vi "stage-controller.vi"() -> ()   [LabVIEW 2014]
uses:
  Stage SubVis/Move stage command - Global - SubVI.ctl
  Stage SubVis/user event out globals - SubVI.vi
  lib/Madlib/Madlib.lvlib
panel:
  out "Current Z (um)":ext
  out "Current Y (um)":ext
  out "Current X (um)":ext
  in  "Curr. Z":dbl(slide) scale=0.0..1.0
  out "Current (X,Y)":cluster{ext[], ext[]}(graph)
  out "At limit 3":bool
  out "At limit 2":bool
  out "At limit":bool
  in  "x,y step (um)":ext=10.0 format="%_5g"
  in  "z step (um)":ext=0.1 format="%_5g"
  in  "y-":bool
  in  "x-":bool
  in  "x+":bool
  in  "z-":bool
  in  "z+":bool
  in  "y+":bool
  in  "Reset stage to center\n         (x, y, and z)":bool
  in  "Stop":bool
  out "Z Range (um)":dbl format="%#_13g"
  out "Y Range (um)":dbl format="%#_13g"
  out "X Range (um)":dbl format="%#_13g"
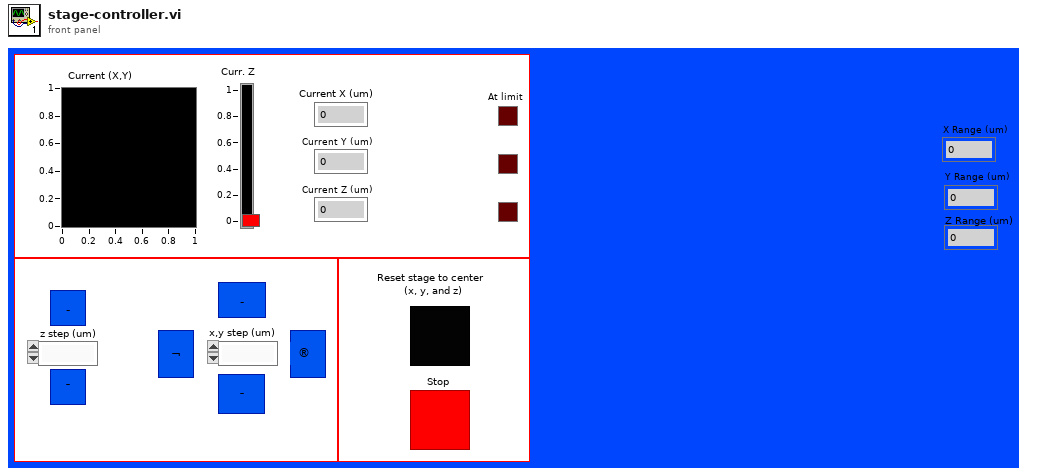
[diagram p1: front panel]
types:
  T1 = cluster{"X Command":dbl, "Y Command":dbl, "Z Command":dbl, "X Position":dbl, "Y Position":dbl, "Z Position":dbl, "X Calibration":dbl, "Y Calibration":dbl, "Z Calibration":dbl}
  T2 = typedef "Move stage command - Global - SubVI.ctl" = cluster{"dx (um) (0 -> ignore)":ext, "dy (um) (0 -> ignore)":ext, "dz (um) (0 -> ignore)":ext, "Re-center x,y":bool, "Re-center z":bool, "x (um) (-1 -> ignore)":dbl, "y (um) (-1 -> ignore)":dbl, "z (um) (-1 -> ignore)":dbl}
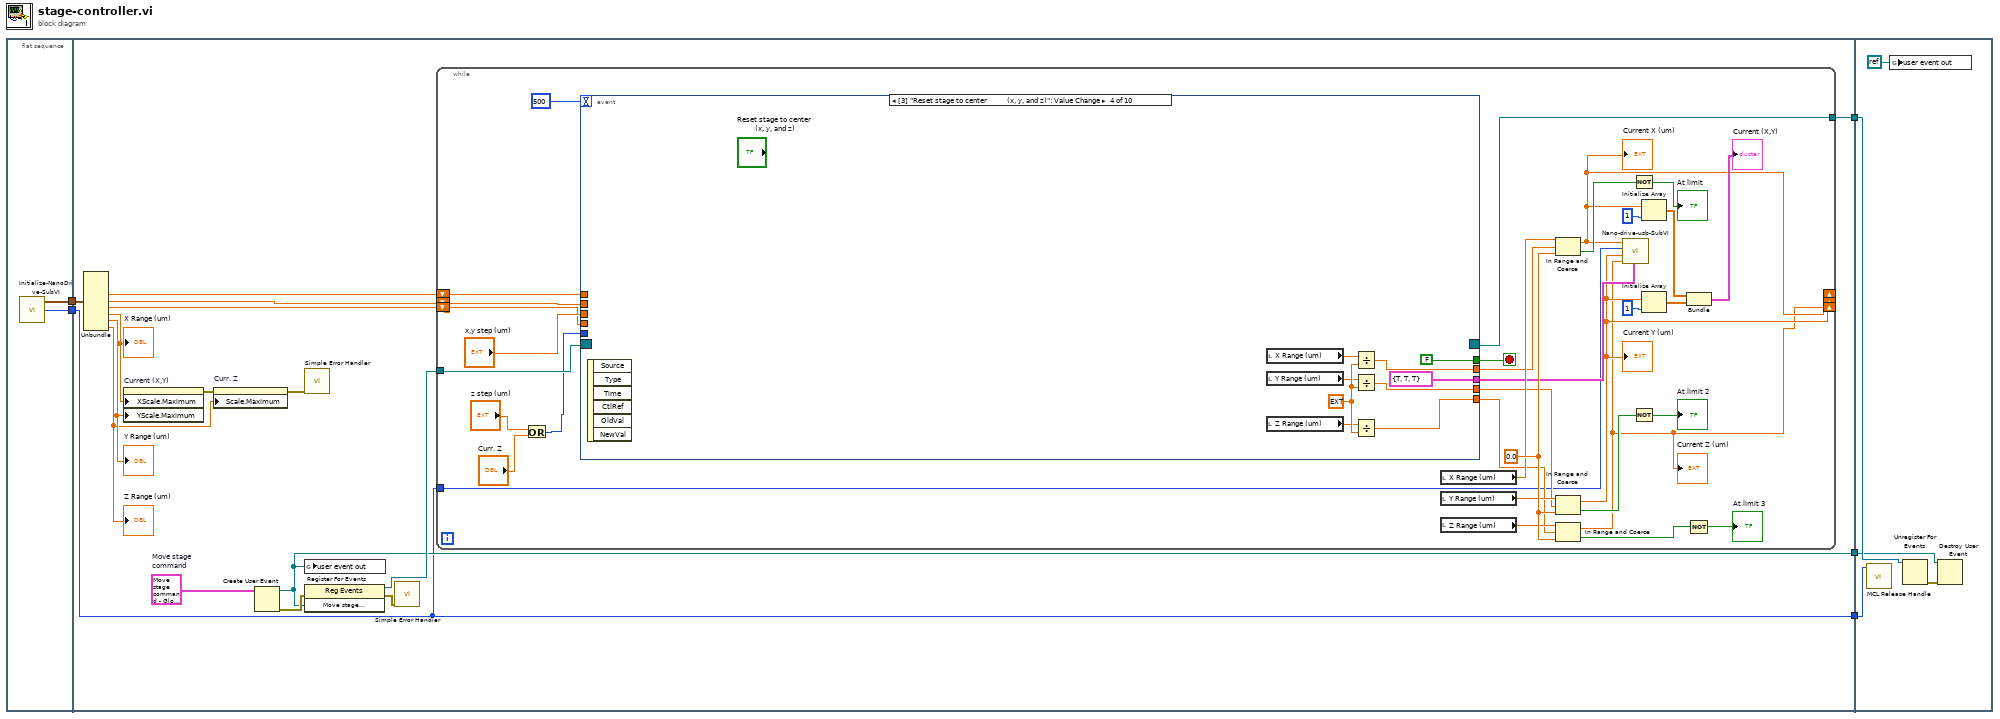
[diagram p0: block diagram]
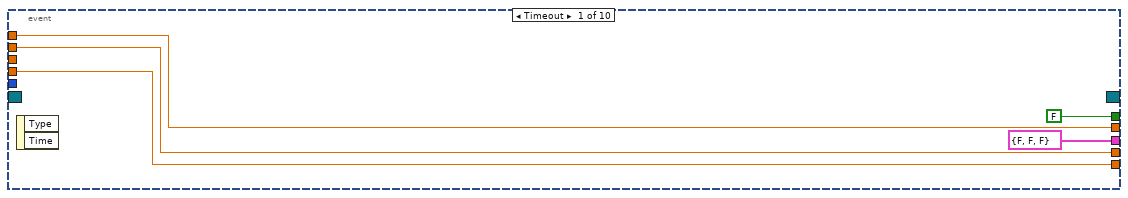
[diagram p2: hidden frame]
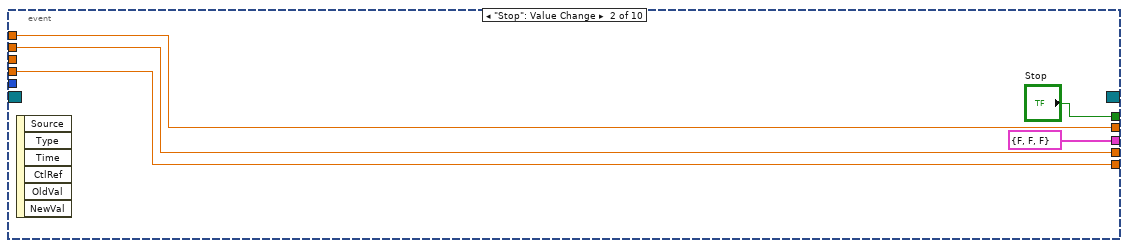
[diagram p3: hidden frame]
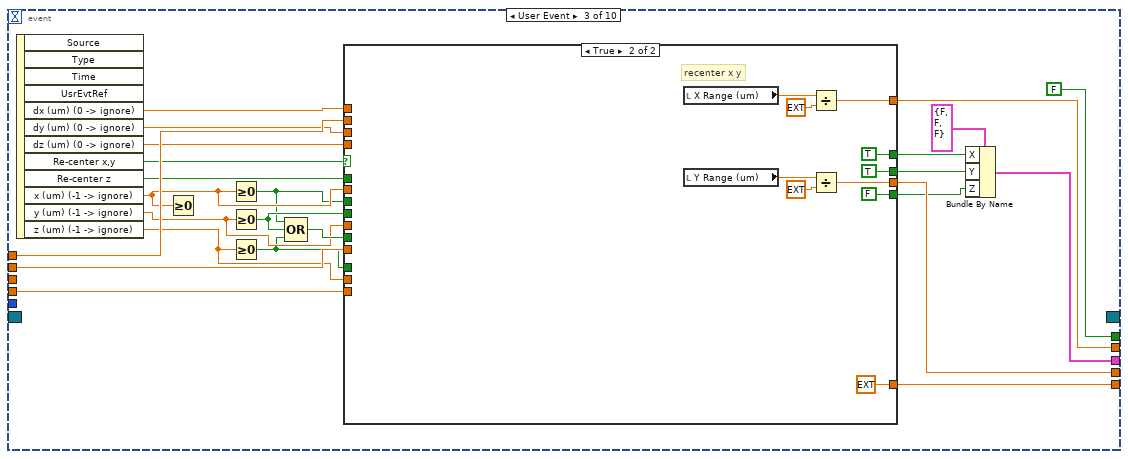
[diagram p4: hidden frame]
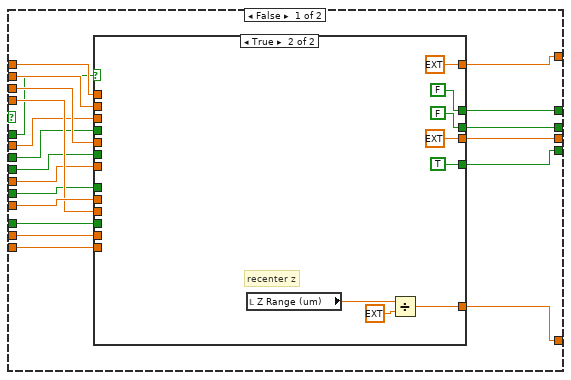
[diagram p5: hidden frame]
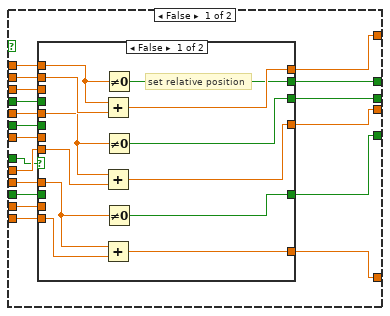
[diagram p6: hidden frame]
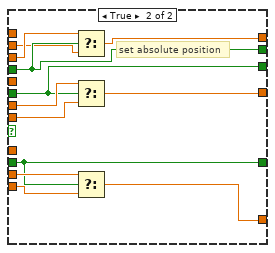
[diagram p7: hidden frame]
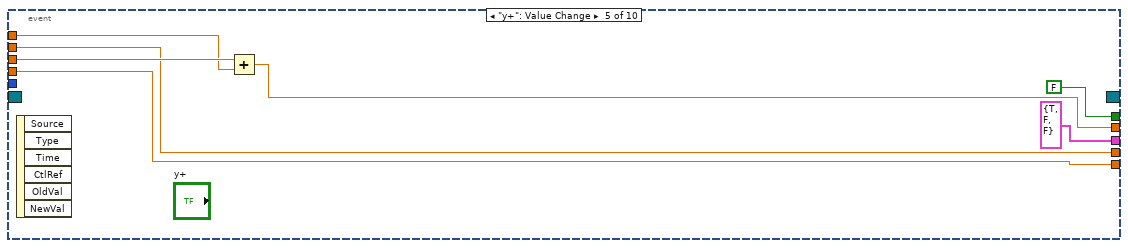
[diagram p8: hidden frame]
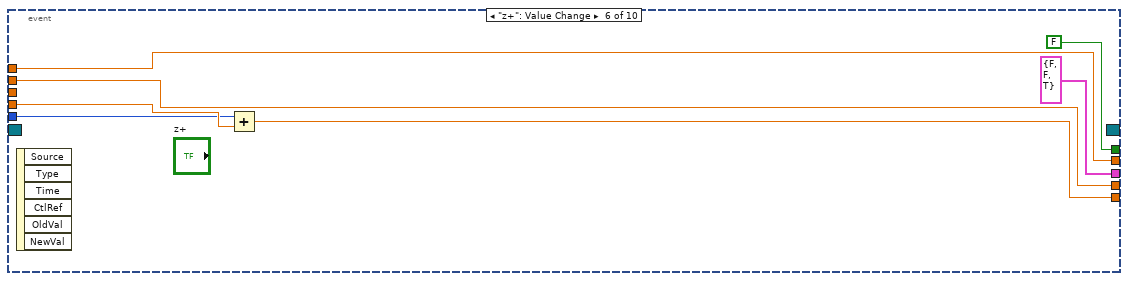
[diagram p9: hidden frame]
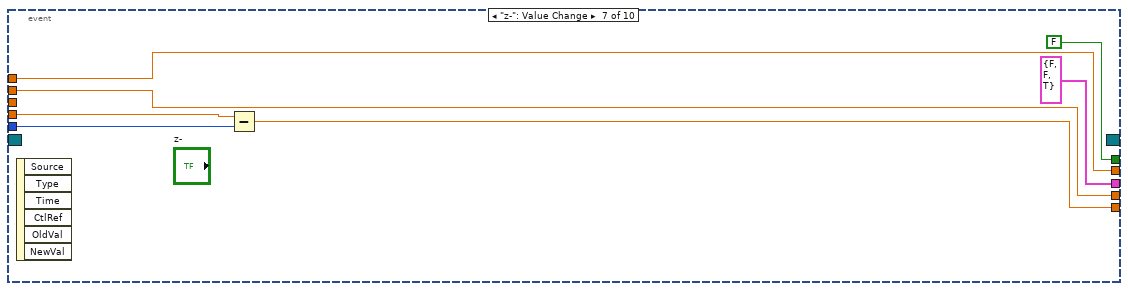
[diagram p10: hidden frame]
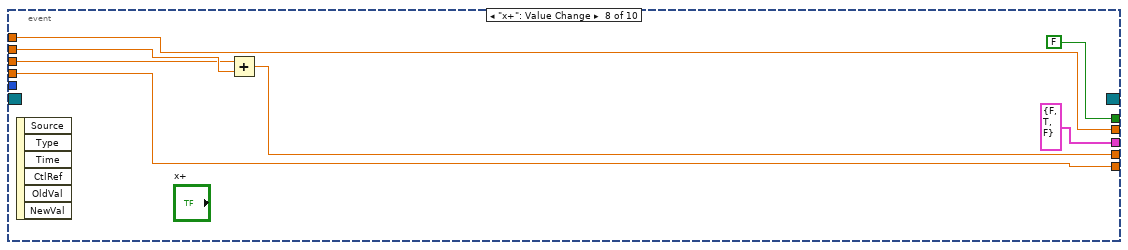
[diagram p11: hidden frame]
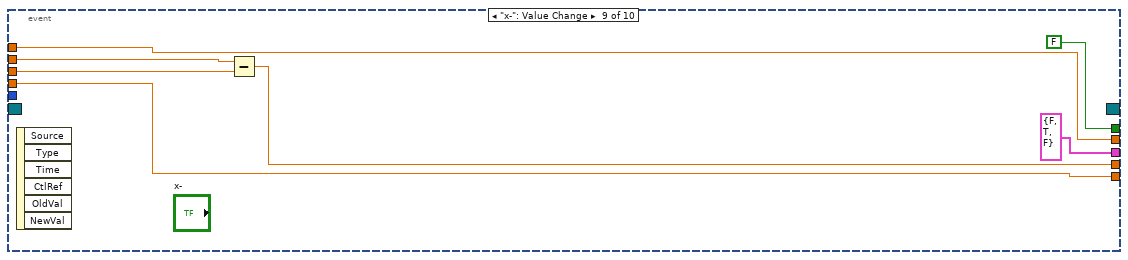
[diagram p12: hidden frame]
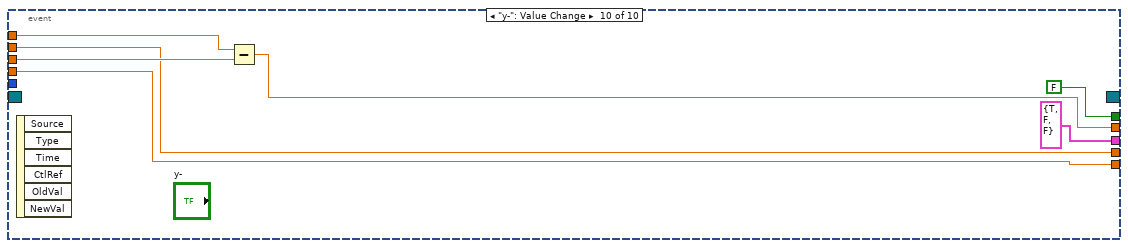
[diagram p13: hidden frame]
diagram:
  n1 = flat-sequence {
    tunnel: [w7] -> w5
    tunnel: [w6] -> w2
    tunnel: w5 -> [w23]
    tunnel: [w18] -> w4
    tunnel: [w17] -> w3
    tunnel: w2 -> [w16]
    tunnel: [w16] -> w1
    tunnel: w4 -> [w227]
    tunnel: w3 -> [w226]
    tunnel: w1 -> [w224]
    frame #0 {
      n2 = call "Initialize-NanoDrive-SubVI.vi"() -> ("Output Pos Info"=w7:T1, "Handle"=w6:i32)  [unwired: 1 in, 1 out]
    }
    frame #1 {
      w22 = T2 {"dx (um) (0 -> ignore)"=0.0, "dy (um) (0 -> ignore)"=0.0, "dz (um) (0 -> ignore)"=0.0, "Re-center x,y"=FALSE, "Re-center z"=FALSE, "x (um) (-1 -> ignore)"=-1.0, "y (um) (-1 -> ignore)"=-1.0, "z (um) (-1 -> ignore)"=-1.0}  # Move stage command
      n3 = Unbundle(w23) -> ("X Position"=w10:dbl, "Y Position"=w9:dbl, "Z Position"=w8:dbl, "X Calibration"=w15:dbl, "Y Calibration"=w14:dbl, "Z Calibration"=w13:dbl)  [unwired: 3 out]
      "Z Range (um)" <- w13
      "Y Range (um)" <- w14
      "X Range (um)" <- w15
      n4 = property on="Current (X,Y)" class="XYGraph (strict)"("XScale.Maximum"=w15, "YScale.Maximum"=w14) -> (error out=w12:errorcluster)  [unwired: 2 in, 1 out]
      n5 = property on="Curr. Z" class="Slide (strict)"(error in=w12, "Scale.Maximum"=w13) -> (error out=w11:errorcluster)  [unwired: 1 in, 1 out]
      n6 = Create User Event(user event datatype=w22) -> (user event=w17:refnum<user-event>, error out=w20:errorcluster)  [unwired: 1 in]
      n7 = call <vilib>:"Simple Error Handler.vi"("error in (no error)"=w11) -> ()  [unwired: 4 in, 5 out]
      n8 = global write "user event out globals - SubVI.vi" "user event out"(w17) -> ()
      n9 = register-events(error in=w20, w17) -> (reference out=w19:refnum<event-registration>, error out=w21:errorcluster)  [unwired: 1 in]
      n10 = call <vilib>:"Simple Error Handler.vi"("error in (no error)"=w21) -> ()  [unwired: 1 in, 8 out]
      n11 = while {
        tunnel: w19 -> [w55]
        tunnel: [w54] -> w18
        tunnel: w16 -> [w33]
        shift-right: [w29] -> _
        shift-left: w10 -> [w32]
        shift-right: [w28] -> _
        shift-left: w9 -> [w31]
        shift-right: [w27] -> _
        shift-left: w8 -> [w30]
        stop <- w56 stop-if-true
        w53 = 0.0
        n12 = Or(x="z step (um)", y="Curr. Z") -> (x .or. y?=w24:i32)
        n13 = event shown="[3] \"Reset stage to center          (x, y, and z)\": Value Change" {
          selector: w55 -> [_ _ _ _ _ _ _ _ _ _]
          dyn-events: [_ _ _ _ _ _ _ _ _ _] -> w54
          timeout: 500 -> [_ _ _ _ _ _ _ _ _ _]
          tunnel: [FALSE ("Stop") "Stop" FALSE ("Stop") FALSE ("Stop") FALSE ("Stop") FALSE ("Stop") FALSE ("Stop") FALSE ("Stop") FALSE ("Stop") FALSE ("Stop")] -> w56
          tunnel: w32 -> [w61 w66 w91 _ w185 w194 w200 w204 w213 w220]
          tunnel: w31 -> [w60 w65 w90 _ w184 w189 w199 w206 w210 w219]
          tunnel: w30 -> [w59 w64 w89 _ w183 w191 w196 w208 w214 w218]
          tunnel: [w61 w66 w86 w176 w187 w194 w200 w204 w213 w222] -> w49
          tunnel: [w60 w65 w87 w179 w184 w189 w199 w207 w215 w219] -> w48
          tunnel: [w59 w64 w88 w178 w183 w193 w202 w208 w214 w218] -> w47
          tunnel: [cluster{"X":bool, "Y":bool, "Z":bool} {"X"=FALSE, "Y"=FALSE, "Z"=FALSE} ("Set this axis?") cluster{"X":bool, "Y":bool, "Z":bool} {"X"=FALSE, "Y"=FALSE, "Z"=FALSE} ("Set this axis?") w79 cluster{"X":bool, "Y":bool, "Z":bool} {"X"=TRUE, "Y"=TRUE, "Z"=TRUE} ("Set this axis?") cluster{"X":bool, "Y":bool, "Z":bool} {"X"=TRUE, "Y"=FALSE, "Z"=FALSE} ("Set this axis?") cluster{"X":bool, "Y":bool, "Z":bool} {"X"=FALSE, "Y"=FALSE, "Z"=TRUE} ("Set this axis?") cluster{"X":bool, "Y":bool, "Z":bool} {"X"=FALSE, "Y"=FALSE, "Z"=TRUE} ("Set this axis?") cluster{"X":bool, "Y":bool, "Z":bool} {"X"=FALSE, "Y"=TRUE, "Z"=FALSE} ("Set this axis?") cluster{"X":bool, "Y":bool, "Z":bool} {"X"=FALSE, "Y"=TRUE, "Z"=FALSE} ("Set this axis?") cluster{"X":bool, "Y":bool, "Z":bool} {"X"=TRUE, "Y"=FALSE, "Z"=FALSE} ("Set this axis?")] -> w34
          tunnel: "x,y step (um)" -> [_ _ _ _ w186 _ _ w205 w211 w221]
          tunnel: w24 -> [_ _ _ _ _ w190 w197 _ _ _]
          event Timeout {
            n14 = event-data() -> ()  [unwired: 3 out]
          }
          event "Stop": Value Change {
            n15 = event-data() -> ()  [unwired: 7 out]
          }
          event User Event {
            n16 = event-data() -> ("dx (um) (0 -> ignore)"=w84:ext, "dy (um) (0 -> ignore)"=w83:ext, "dz (um) (0 -> ignore)"=w82:ext, "Re-center x,y"=w81:bool, "Re-center z"=w75:bool, "x (um) (-1 -> ignore)"=w71:dbl, "y (um) (-1 -> ignore)"=w72:dbl, "z (um) (-1 -> ignore)"=w73:dbl)  [unwired: 5 out]
            n17 = Greater Or Equal To 0?(x=w71) -> ()  [unwired: 1 out]
            n18 = Greater Or Equal To 0?(x=w71) -> (x >= 0?=w68:bool)
            n19 = Greater Or Equal To 0?(x=w72) -> (x >= 0?=w69:bool)
            n20 = Greater Or Equal To 0?(x=w73) -> (x >= 0?=w70:bool)
            n21 = Compound Arithmetic op=OR(w68, w69, w70) -> (w74:bool)
            n22 = case shown="True" w81 {
              tunnel: w91 -> [w111 _]
              tunnel: w90 -> [w110 _]
              tunnel: w89 -> [w109 _]
              tunnel: [w108 ext 0.0] -> w88
              tunnel: [w107 w165] -> w87
              tunnel: [w106 w167] -> w86
              tunnel: w84 -> [w105 _]
              tunnel: w83 -> [w104 _]
              tunnel: w82 -> [w103 _]
              tunnel: [w102 FALSE] -> w78
              tunnel: [w101 TRUE] -> w77
              tunnel: [w100 TRUE] -> w76
              tunnel: w75 -> [w99 _]
              tunnel: w74 -> [w98 _]
              tunnel: w73 -> [w97 _]
              tunnel: w72 -> [w96 _]
              tunnel: w71 -> [w95 _]
              tunnel: w70 -> [w94 _]
              tunnel: w69 -> [w93 _]
              tunnel: w68 -> [w92 _]
              frame False {
                n23 = case shown="True" w99 {
                  tunnel: w111 -> [w130 _]
                  tunnel: w110 -> [w129 _]
                  tunnel: w109 -> [w128 _]
                  tunnel: [w127 w161] -> w108
                  tunnel: [w126 ext 0.0] -> w107
                  tunnel: [w125 ext 0.0] -> w106
                  tunnel: w105 -> [w124 _]
                  tunnel: w104 -> [w123 _]
                  tunnel: w103 -> [w122 _]
                  tunnel: [w121 TRUE] -> w102
                  tunnel: [w120 FALSE] -> w101
                  tunnel: [w119 FALSE] -> w100
                  tunnel: w98 -> [w118 _]
                  tunnel: w97 -> [w117 _]
                  tunnel: w96 -> [w116 _]
                  tunnel: w95 -> [w115 _]
                  tunnel: w94 -> [w114 _]
                  tunnel: w93 -> [w113 _]
                  tunnel: w92 -> [w112 _]
                  frame False {
                    n24 = case shown="False" w118 {
                      tunnel: w130 -> [w142 w150]
                      tunnel: w129 -> [w141 w147]
                      tunnel: w128 -> [w140 w144]
                      tunnel: [w139 w146] -> w127
                      tunnel: [w138 w149] -> w126
                      tunnel: [w137 w153] -> w125
                      tunnel: w124 -> [w136 _]
                      tunnel: w123 -> [w135 _]
                      tunnel: w122 -> [w134 _]
                      tunnel: [w133 w143] -> w121
                      tunnel: [w132 w148] -> w120
                      tunnel: [w131 w152] -> w119
                      tunnel: w117 -> [_ w145]
                      tunnel: w116 -> [_ w154]
                      tunnel: w115 -> [_ w151]
                      tunnel: w114 -> [_ w143]
                      tunnel: w113 -> [_ w148]
                      tunnel: w112 -> [_ w152]
                      frame False {
                        # "set relative position"
                        n25 = Add(x=w136, y=w142) -> (x+y=w137:ext)
                        n26 = Add(x=w135, y=w141) -> (x+y=w138:ext)
                        n27 = Add(x=w134, y=w140) -> (x+y=w139:ext)
                        n28 = Not Equal To 0?(x=w136) -> (x != 0?=w131:bool)
                        n29 = Not Equal To 0?(x=w135) -> (x != 0?=w132:bool)
                        n30 = Not Equal To 0?(x=w134) -> (x != 0?=w133:bool)
                      }
                      frame True {
                        # "set absolute position"
                        n31 = Select(t=w151, s=w152, f=w150) -> (s? t:f=w153:ext)
                        n32 = Select(t=w154, s=w148, f=w147) -> (s? t:f=w149:ext)
                        n33 = Select(t=w145, s=w143, f=w144) -> (s? t:f=w146:ext)
                      }
                    }
                  }
                  frame True {
                    # "recenter z"
                    n34 = local read "Z Range (um)"() -> (w155:dbl)
                    n35 = Divide(x=w155, y=ext 2.0) -> (x/y=w161:ext)
                  }
                }
              }
              frame True {
                # "recenter x y"
                n36 = local read "X Range (um)"() -> (w164:dbl)
                n37 = local read "Y Range (um)"() -> (w163:dbl)
                n38 = Divide(x=w164, y=ext 2.0) -> (x/y=w167:ext)
                n39 = Divide(x=w163, y=ext 2.0) -> (x/y=w165:ext)
              }
            }
            n40 = Bundle By Name(cluster=cluster{"X":bool, "Y":bool, "Z":bool} {"X"=FALSE, "Y"=FALSE, "Z"=FALSE} ("Set this axis?"), "X"=w76, "Y"=w77, "Z"=w78) -> (w79:cluster{"X":bool, "Y":bool, "Z":bool})
          }
          event "Reset stage to center\n         (x, y, and z)": Value Change {
            w177 = ext 2.0 ("y")
            n41 = event-data() -> ()  [unwired: 7 out]
            n42 = local read "X Range (um)"() -> (w173:dbl)
            n43 = local read "Y Range (um)"() -> (w174:dbl)
            n44 = local read "Z Range (um)"() -> (w175:dbl)
            n45 = Divide(x=w173, y=w177) -> (x/y=w176:ext)
            n46 = Divide(x=w174, y=w177) -> (x/y=w179:ext)
            n47 = Divide(x=w175, y=w177) -> (x/y=w178:ext)
          }
          event "y+": Value Change {
            n48 = event-data() -> ()  [unwired: 7 out]
            n49 = Add(x=w186, y=w185) -> (x+y=w187:ext)
          }
          event "z+": Value Change {
            n50 = event-data() -> ()  [unwired: 7 out]
            n51 = Add(x=w190, y=w191) -> (x+y=w193:ext)
          }
          event "z-": Value Change {
            n52 = event-data() -> ()  [unwired: 7 out]
            n53 = Subtract(x=w196, y=w197) -> (x-y=w202:ext)
          }
          event "x+": Value Change {
            n54 = event-data() -> ()  [unwired: 7 out]
            n55 = Add(x=w205, y=w206) -> (x+y=w207:ext)
          }
          event "x-": Value Change {
            n56 = event-data() -> ()  [unwired: 7 out]
            n57 = Subtract(x=w210, y=w211) -> (x-y=w215:ext)
          }
          event "y-": Value Change {
            n58 = event-data() -> ()  [unwired: 7 out]
            n59 = Subtract(x=w220, y=w221) -> (x-y=w222:ext)
          }
        }
        n60 = local read "X Range (um)"() -> (w51:dbl)
        n61 = local read "Y Range (um)"() -> (w52:dbl)
        n62 = local read "Z Range (um)"() -> (w50:dbl)
        n63 = In Range and Coerce(upper limit=w51, x=w49, lower limit=w53) -> (coerced(x)=w29:ext, In Range?=w45:bool)
        "Current X (um)" <- w29
        n64 = In Range and Coerce(upper limit=w52, x=w48, lower limit=w53) -> (coerced(x)=w28:ext, In Range?=w43:bool)
        "Current Y (um)" <- w28
        n65 = In Range and Coerce(upper limit=w50, x=w47, lower limit=w53) -> (coerced(x)=w27:ext, In Range?=w41:bool)
        "Current Z (um)" <- w27
        n66 = call "Nano-drive-usb-SubVI.vi"("Set this axis?"=w34, "Z (um)"=w27, "Y (um)"=w28, "Numeric"=w33, "X (um)"=w29) -> ()  [unwired: 6 in]
        n67 = Not(x=w45) -> (.not. x?=→"At limit":bool)
        n68 = Not(x=w43) -> (.not. x?=→"At limit 2":bool)
        n69 = Initialize Array(w29, 1) -> (w37:ext[])
        n70 = Initialize Array(w28, 1) -> (w36:ext[])
        n71 = Bundle(w37, w36) -> (→"Current (X,Y)":cluster{ext[], ext[]})  [unwired: 1 out]
        n72 = Not(x=w41) -> (.not. x?=→"At limit 3":bool)
      }
    }
    frame #2 {
      n73 = call "MCL Release Handle.vi"("handle"=w224) -> ()  [unwired: 10 in, 1 out]
      n74 = global write "user event out globals - SubVI.vi" "user event out"(refnum<k0> refnum) -> ()
      n75 = Unregister For Events(event registration refnum=w227) -> (error out=w228:errorcluster)  [unwired: 1 in]
      n76 = Destroy User Event(user event=w226, error in=w228) -> ()  [unwired: 1 out]
    }
  }
